vi "Correlation_Profile.vi"(4 "Point Increment In":i32, 5 "Loop i":i32, 6 "Arguments":string[](array[string]), 7 "Simulate/Run":T1) -> (0 "Point Increment Out":i32, 1 "Point index":i32, 2 "Error String":string, 3 "Continue":bool)   [LabVIEW 2022 SP3]
uses:
  Controls/User_Specific_mode.ctl
  Globals/Dynamic_call_global.ph.vi
panel:
  out "Current Value":dbl
  out "Max correlation":dbl
  out "Absolute Value":dbl
  out "Desired Value":dbl
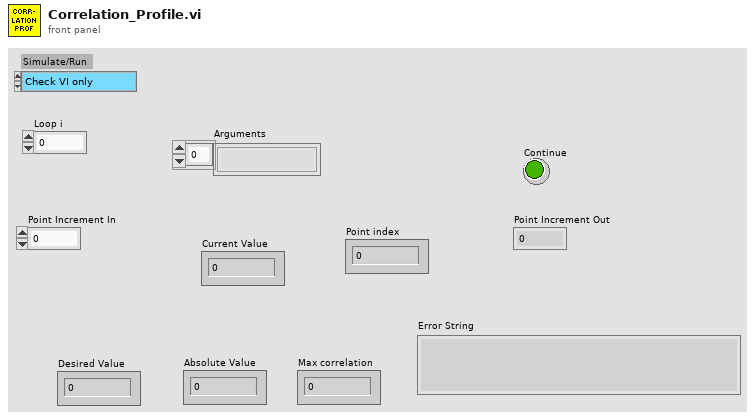
[diagram p1: front panel]
types:
  T1 = typedef "User_Specific_mode.ctl" = enum16{"Check VI only", "Run VI"}
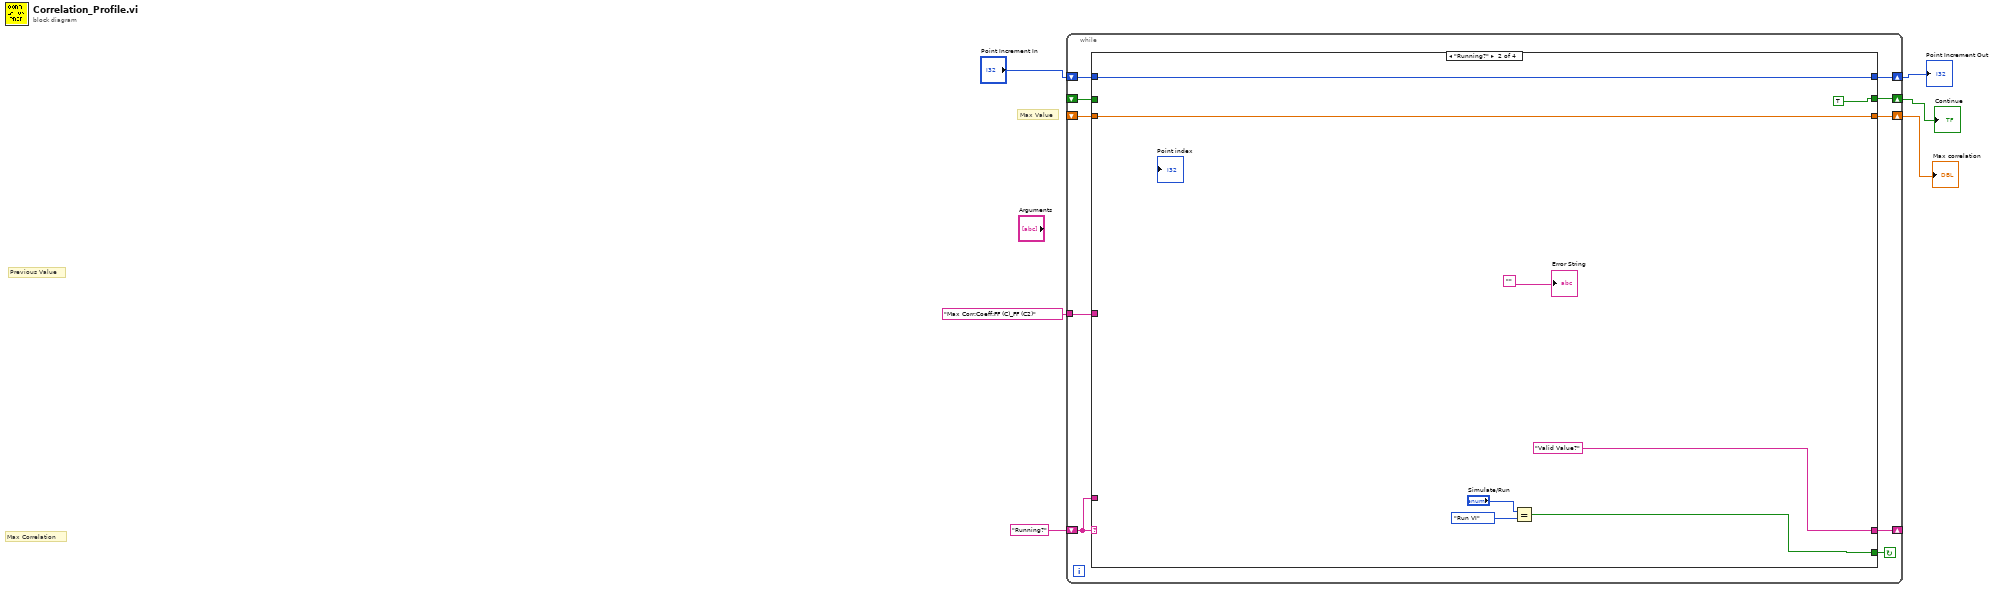
[diagram p0: block diagram]
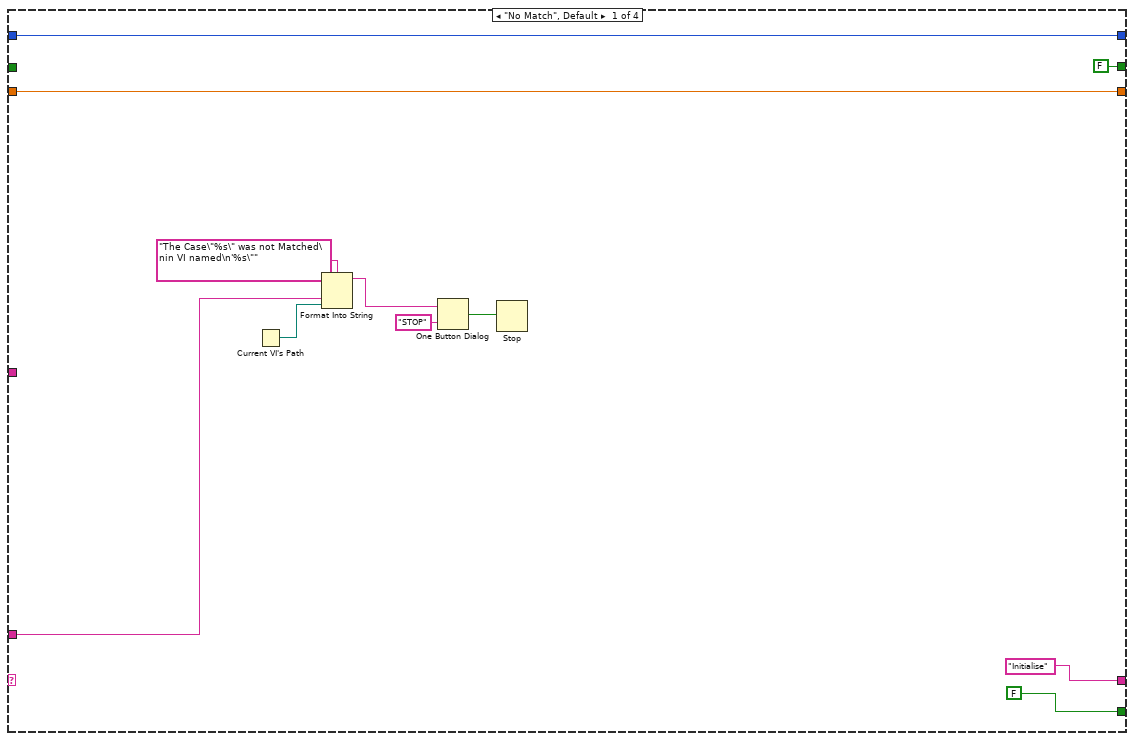
[diagram p2: hidden frame]
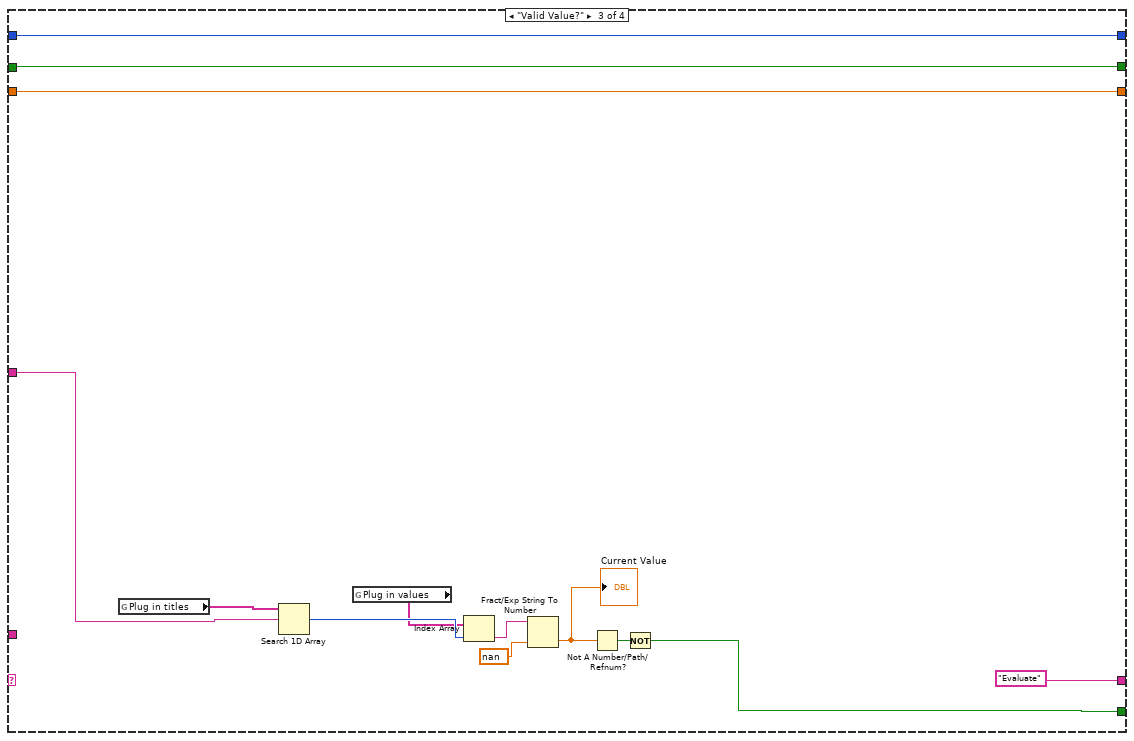
[diagram p3: hidden frame]
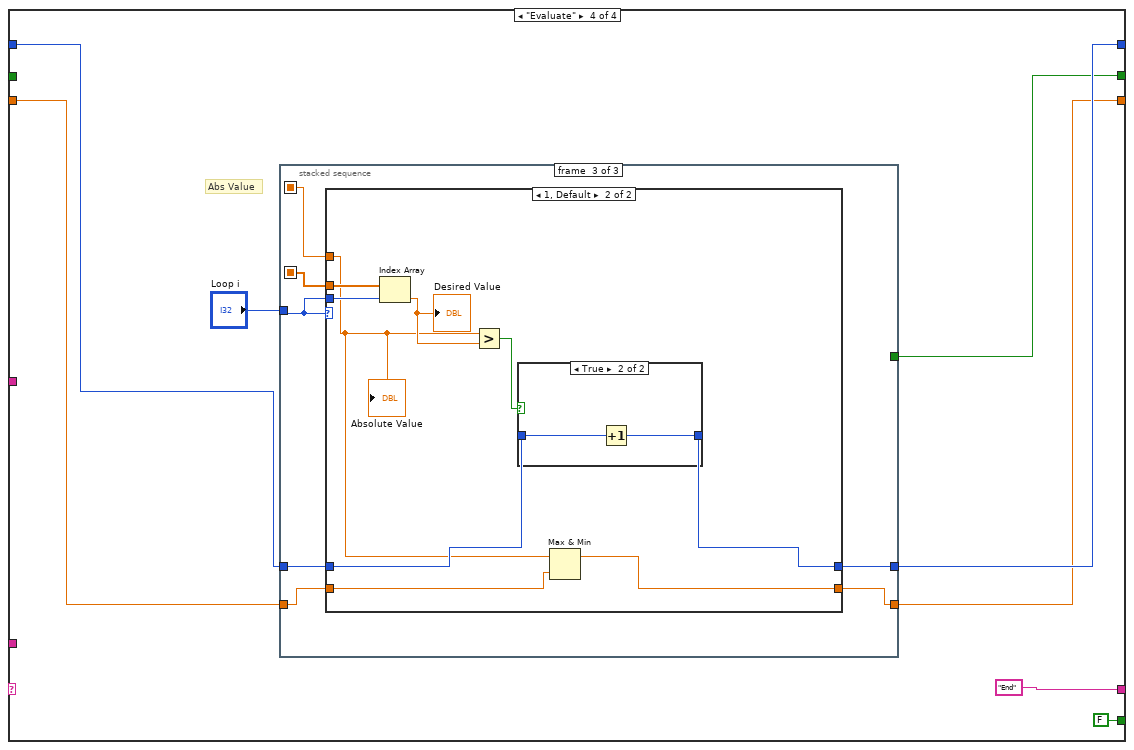
[diagram p4: hidden frame]
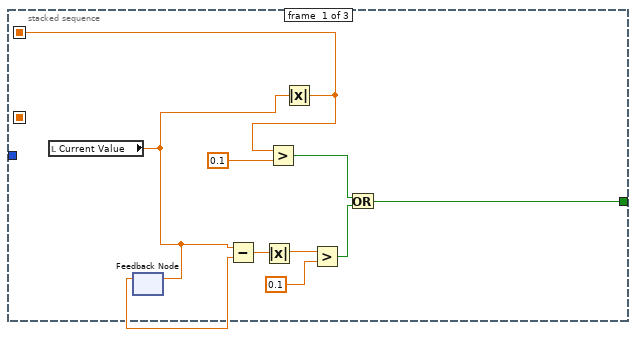
[diagram p5: hidden frame]
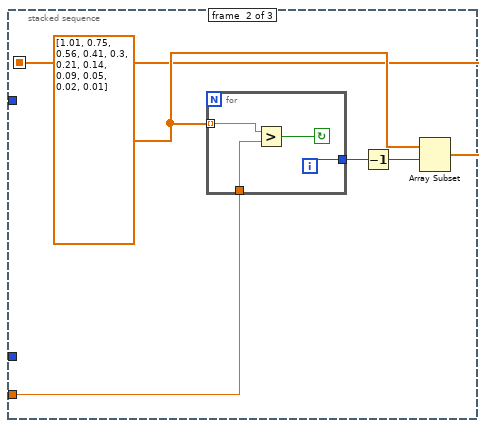
[diagram p6: hidden frame]
diagram:
  # "Max Value"
  # "Previous Value"
  # "Max Correlation"
  n1 = while {
    shift-left: "Running?" -> [w14]
    shift-right: [w15] -> _
    shift-right: [w12] -> w4
    shift-left: "Point Increment In" -> [w13]
    shift-right: [w11] -> w2
    shift-left: _ -> [w10]
    shift-right: [w9] -> w3
    shift-left: _ -> [w8]
    tunnel: "Max Corr:Coeff:FF (C)_FF (C2)" -> [w7]
    stop <- w16 continue-if-true
    n2 = case shown="\"Running?\"" w14 {
      tunnel: [FALSE w32 w40 FALSE] -> w16
      tunnel: ["Initialise" "Valid Value?" "Evaluate" "End"] -> w15
      tunnel: w14 -> [w22 _ _ _]
      tunnel: w13 -> [w19 w31 w38 w54]
      tunnel: [w19 w31 w38 w53] -> w12
      tunnel: [FALSE TRUE w39 w52] -> w11
      tunnel: w10 -> [_ _ w39 _]
      tunnel: [w17 w29 w37 w51] -> w9
      tunnel: w8 -> [w17 w29 w37 w50]
      tunnel: w7 -> [_ _ w36 _]
      frame "No Match", Default {
        n3 = Current VI's Path() -> (path=w21:path)
        n4 = Format Into String(format string="The Case\"%s\" was not Matched\nin VI named\n'%s\"" ("Format String"), w22, w21) -> (resulting string=w25:string)  [unwired: 2 in, 1 out]
        n5 = One Button Dialog(message=w25, button name ("OK")="STOP") -> (true=w23:bool)
        n6 = Stop(stop? (T)=w23) -> ()
      }
      frame "Running?" {
        n7 = Equal?(x="Simulate/Run", y=User_Specific_mode."Run VI" ("Simulate/Run")) -> (x = y?=w32:bool)
        "Error String" <- ""
      }
      frame "Valid Value?" {
        n8 = global read "Dynamic_call_global.ph.vi" "Plug in titles"() -> (w42:string[])
        n9 = Search 1D Array(1D array=w42, element=w36) -> (index of element=w45:i32)  [unwired: 1 in]
        n10 = global read "Dynamic_call_global.ph.vi" "Plug in values"() -> (w44:string[])
        n11 = Index Array(array=w44, index=w45) -> (element=w43:string)
        n12 = Fract/Exp String To Number(string=w43, default (0 dbl)=nan ("default (0 DBL)")) -> (number=w47:dbl)  [unwired: 2 in, 1 out]
        "Current Value" <- w47
        n13 = Not A Number/Path/Refnum?(number/path/refnum=w47) -> (NaN/Path/Refnum?=w41:bool)
        n14 = Not(x=w41) -> (.not. x?=w40:bool)
      }
      frame "Evaluate" {
        # "Abs Value"
        n15 = stacked-sequence {
          seq-local: [w59 _ _] -> [_ _ w82]
          seq-local: [_ w68 _] -> [_ _ w76]
          tunnel: [w60 _ _] -> w52
          tunnel: "Loop i" -> [_ _ w77]
          tunnel: [_ _ w81] -> w51
          tunnel: w50 -> [_ w71 w80]
          tunnel: [_ _ w79] -> w53
          tunnel: w54 -> [_ _ w78]
          frame #0 {
            n16 = local read "Current Value"() -> (w57:dbl)
            n17 = feedback-in #1(w57) -> ()
            n18 = feedback #1() -> (w58:dbl)  [unwired: 1 in]
            n19 = Subtract(x=w57, y=w58) -> (x-y=w65:dbl)
            n20 = Absolute Value(x=w65) -> (abs(x)=w64:dbl)
            n21 = Absolute Value(x=w57) -> (abs(x)=w59:dbl)
            n22 = Greater?(x=w59, y=0.1) -> (0:w61:bool)
            n23 = Greater?(x=w64, y=0.1) -> (0:w62:bool)
            n24 = Or(x=w61, y=w62) -> (x .or. y?=w60:bool)
          }
          frame #1 {
            w69 = dbl[] [1.01, 0.75, 0.56, 0.41, 0.3, 0.21, 0.14, 0.09, 0.05, 0.02, 0.01]
            n25 = for {
              tunnel: w69 -> [w75] mode=indexing
              tunnel: w71 -> [w74]
              tunnel: [w72] -> w70
              i -> [w72]
              stop <- w73 continue-if-true
              n26 = Greater?(x=w75, y=w74) -> (0:w73:bool)
            }
            n27 = Decrement(x=w70) -> (x-1=w67:i32)
            n28 = Array Subset(array=w69, index=w67) -> (w68:dbl[])  [unwired: 1 in]
          }
          frame #2 {
            n29 = case shown="1, Default" w77 {
              tunnel: w82 -> [w83 w86]
              tunnel: [w83 w85] -> w81
              tunnel: w80 -> [_ w87]
              tunnel: [w84 w91] -> w79
              tunnel: w78 -> [w84 w92]
              tunnel: w77 -> [_ w93]
              tunnel: w76 -> [_ w89]
              frame 0 {
              }
              frame 1, Default {
                n30 = Index Array(array=w89, index=w93) -> (element=w88:dbl)
                "Desired Value" <- w88
                n31 = Greater?(x=w86, y=w88) -> (0:w90:bool)
                n32 = case shown="True" w90 {
                  tunnel: w92 -> [w94 w96]
                  tunnel: [w94 w95] -> w91
                  frame False {
                  }
                  frame True {
                    n33 = Increment(x=w96) -> (x+1=w95:i32)
                  }
                }
                n34 = Max & Min(x=w86, y=w87) -> (max(x,y)=w85:dbl)  [unwired: 1 out]
                "Absolute Value" <- w86
              }
            }
          }
        }
      }
    }
  }
  "Point Increment Out" <- w4
  "Continue" <- w2
  "Max correlation" <- w3
